vi "test Connect.vi"(8 "error in (no error)":errorcluster, 11 "TestCase in":refnum<class "Test Data Stream.lvclass">) -> (0 "error out":errorcluster, 3 "TestCase out":refnum<class "Test Data Stream.lvclass">)   [LabVIEW 2020, in "Test Data Stream.lvclass"]
uses:
  Test Data Stream.lvclass
  <vilib>/addons/_JKI Toolkits/VI Tester/TestCase.llb/TestCase.lvclass
  Source/Protocols/TCP Strategy/TCP Stream/TCP Stream.lvclass
  C:/Program Files (x86)/National Instruments/LabVIEW 2021/vi.lib/addons/_JKI Toolkits/VI Tester/TestCase.llb/TestCase.lvclass
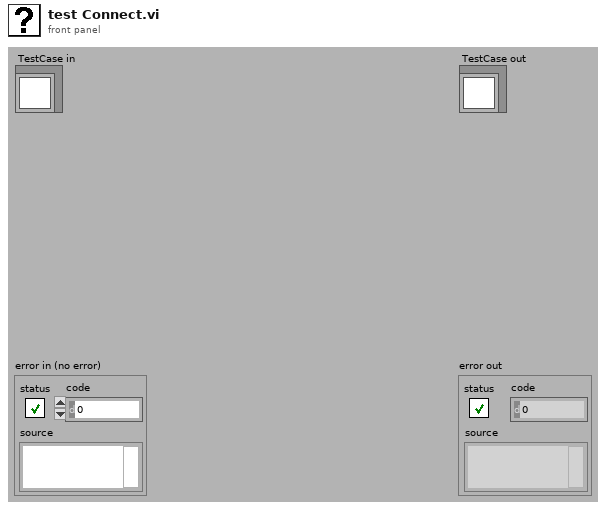
[diagram p1: front panel]
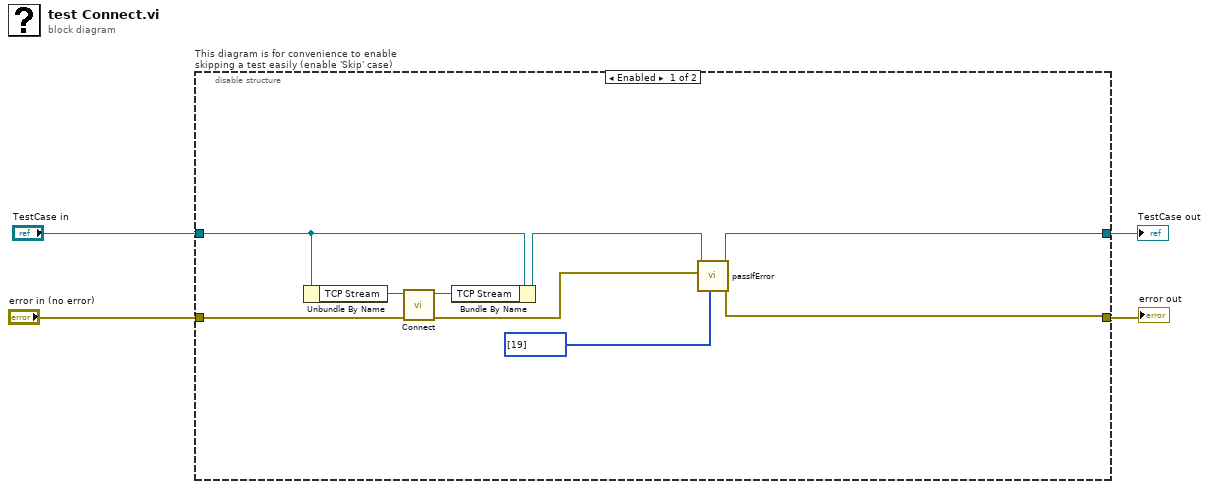
[diagram p0: block diagram]
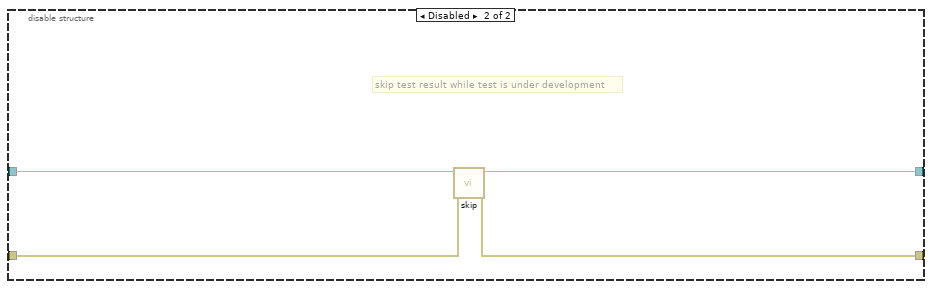
[diagram p2: hidden frame]
diagram:
  n1 = disable-structure "This diagram is for convenience to enable skipping a test easily (enable 'Skip' case)" shown="Enabled" {
    disable-tunnel: "TestCase in" -> [w6 w17]
    disable-tunnel: [w13 w15] -> w1
    disable-tunnel: [w12 w16] -> w3
    disable-tunnel: "error in (no error)" -> [w11 w14]
    frame Enabled {
      n2 = Unbundle By Name(w6) -> ("TCP Stream"=w8:refnum<class "TCP Stream.lvclass">)
      n3 = call-dynamic "Connect.vi"("error in (no error)"=w11, "Message Stream in"=w8) -> ("error out"=w10:errorcluster, "Message Stream out"=w7:refnum<class "TCP Stream.lvclass">)  [unwired: 8 in]
      n4 = Bundle By Name(cluster=w6, "TCP Stream"=w7) -> (w5:refnum<class "Test Data Stream.lvclass">)
      n5 = call-dynamic "passIfError.vi"("passing error codes (default = any error code)"=i32[] [19], "error"=w10, "TestCase in"=w5) -> ("error out"=w12:errorcluster, "TestCase out"=w13:refnum<class "Test Data Stream.lvclass">)  [unwired: 7 in]
    }
    frame Disabled {
      # "skip test result while test is under development"
      n6 = call <vilib>:"skip.vi"("error in (no error)"=w14, "TestCase in"=w17) -> ("error out"=w16:errorcluster, "TestCase out"=w15:refnum<class "Test Data Stream.lvclass">)  [unwired: 8 in]
    }
  }
  "error out" <- w3
  "TestCase out" <- w1
